vi "Timing Engine.vi"(8 "error in (no error)":errorcluster, 9 "Time Limit":dbl, 10 "Reset Time":bool, 11 "Advance Time":bool) -> (0 "error out":errorcluster, 2 "Time Expired?":bool, 3 "Elapsed Time":dbl)   [LabVIEW 2021]
doc: "This Functional Global is helpful for doing timing. It can be reset, advanced, or paused and features a time limit input"
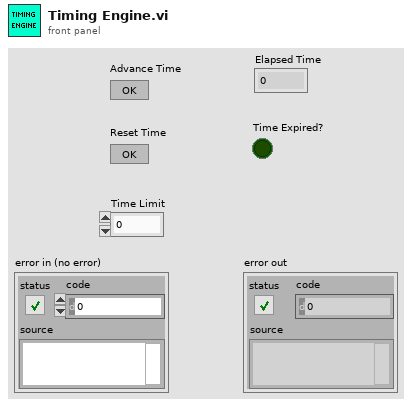
[diagram p1: front panel]
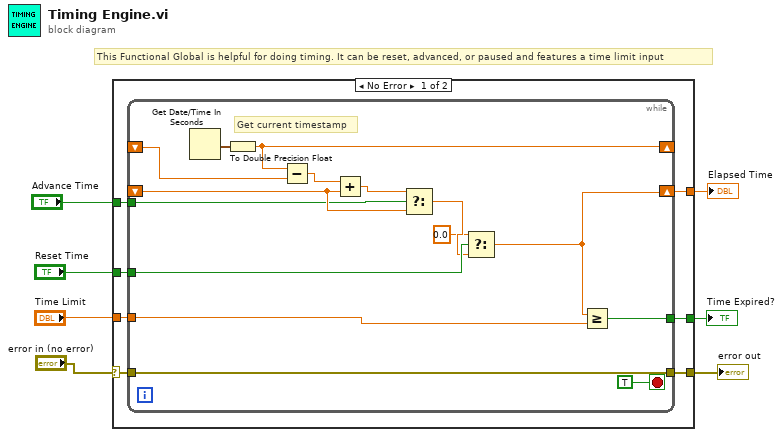
[diagram p0: block diagram]
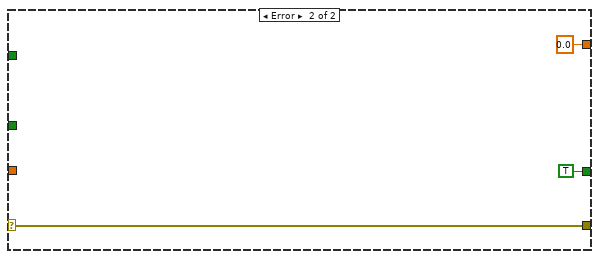
[diagram p2: hidden frame]
diagram:
  # "This Functional Global is helpful for doing timing. It can be reset, advanced, or paused and features a time limit input"
  n1 = case shown="No Error" "error in (no error)" {
    selector: "error in (no error)" -> [w9 w32]
    tunnel: "Advance Time" -> [w14 _]
    tunnel: "Reset Time" -> [w13 _]
    tunnel: "Time Limit" -> [w12 _]
    tunnel: [w11 0.0 ("t")] -> w4
    tunnel: [w10 TRUE] -> w3
    tunnel: [w8 w32] -> w1
    frame No Error {
      n2 = while {
        shift-right: [w27] -> _
        shift-left: _ -> [w26]
        shift-right: [w17] -> w11
        shift-left: _ -> [w23]
        tunnel: w14 -> [w22]
        tunnel: w13 -> [w21]
        tunnel: w12 -> [w18]
        tunnel: [w16] -> w10
        tunnel: [w15] -> w8
        tunnel: w9 -> [w15]
        stop <- TRUE stop-if-true
        # "Get current timestamp"
        n3 = Get Date/Time In Seconds() -> (seconds since 1Jan1904=w28:timestamp)
        n4 = To Double Precision Float(number=w28) -> (double precision float=w27:dbl)
        n5 = Subtract(x=w27, y=w26) -> (x-y=w25:dbl)
        n6 = Add(x=w25, y=w23) -> (x+y=w24:dbl)
        n7 = Select(t=w24, s=w22, f=w23) -> (s? t:f=w20:dbl)
        n8 = Select(t=0.0, s=w21, f=w20) -> (s? t:f=w17:dbl)
        n9 = Greater Or Equal?(x=w17, y=w18) -> (x >= y?=w16:bool)
      }
    }
    frame Error {
    }
  }
  "Time Expired?" <- w3
  "Elapsed Time" <- w4
  "error out" <- w1
